vi "Measurement UI.vi"() -> ()   [LabVIEW 2021, in "ImageRendering.lvlib"]
uses:
  ImageRendering.lvlib
  <vilib>/vision/Image Controls.llb/IMAQ Image.ctl
  nivision.dll
  nivissvc.dll
panel:
  out "Average Time to receive image frame":dbl
  out "Time taken to receive image frame":dbl
  out "Image Acq time":string
  out "Display Frames per Second (approx)":u32
  out "Last Buffer Number":u32
  out "Time to convert back to Image (s)":dbl
  in  "Border Size":i32=3
  in  "Image Name":string="copy"
  in  "Image Type":u32(ring)=4 items=["Grayscale (U8)", "Grayscale (I16)", "Grayscale (SGL)", "Complex (CSG)", "RGB (U32)", "HSL (U32)", "RGB (U64)", "Grayscale (U16)"]
  out "Image Resolution":i32[](array[numeric])
  in  "Camera name":string
  out "Image Pixels (U32)":u32[](array[numeric])
  in  "Image Pixels (U64) 2":T1[][](array[typedef])
  in  "Image Converison Type":string(combo)="ImagePixelArray"
  out "Image Data Received":string
  out "value":u32[][](array[numeric])
  out "Image":T2(plugin-control)
  out "error out":errorcluster
  out "Image Data":string
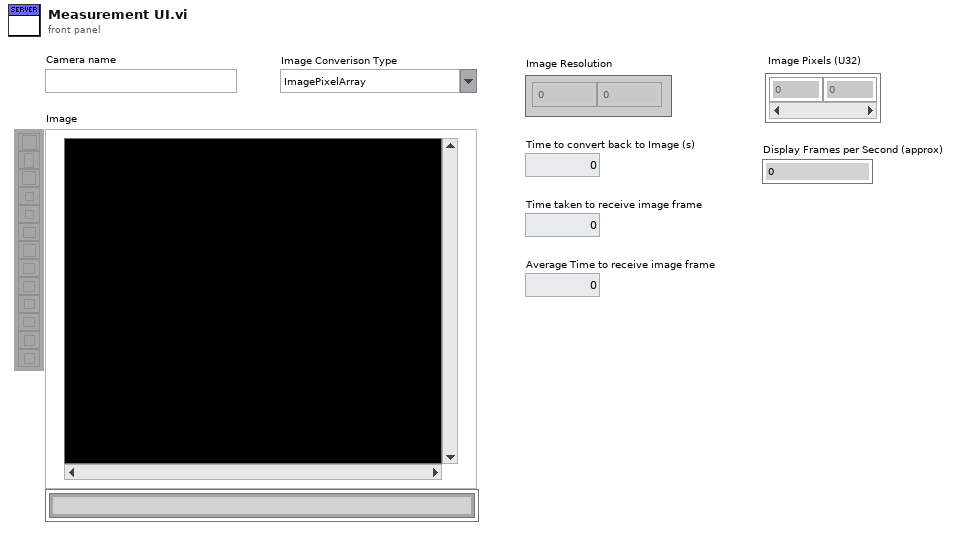
[diagram p1: front panel]
types:
  T1 = typedef "Color (U64)" = cluster{"Plane 3 (Blue)":u16, "Plane 2 (Green)":u16, "Plane 1 (Red)":u16, "Plane 4 (alpha)":u16}
  T2 = typedef "IMAQ Image.ctl" = refnum<image>
  T3 = cluster{"New Image":T2, "Run start time":timestamp, "Last Buffer Number":u32, "Time to receive image":dbl[]}
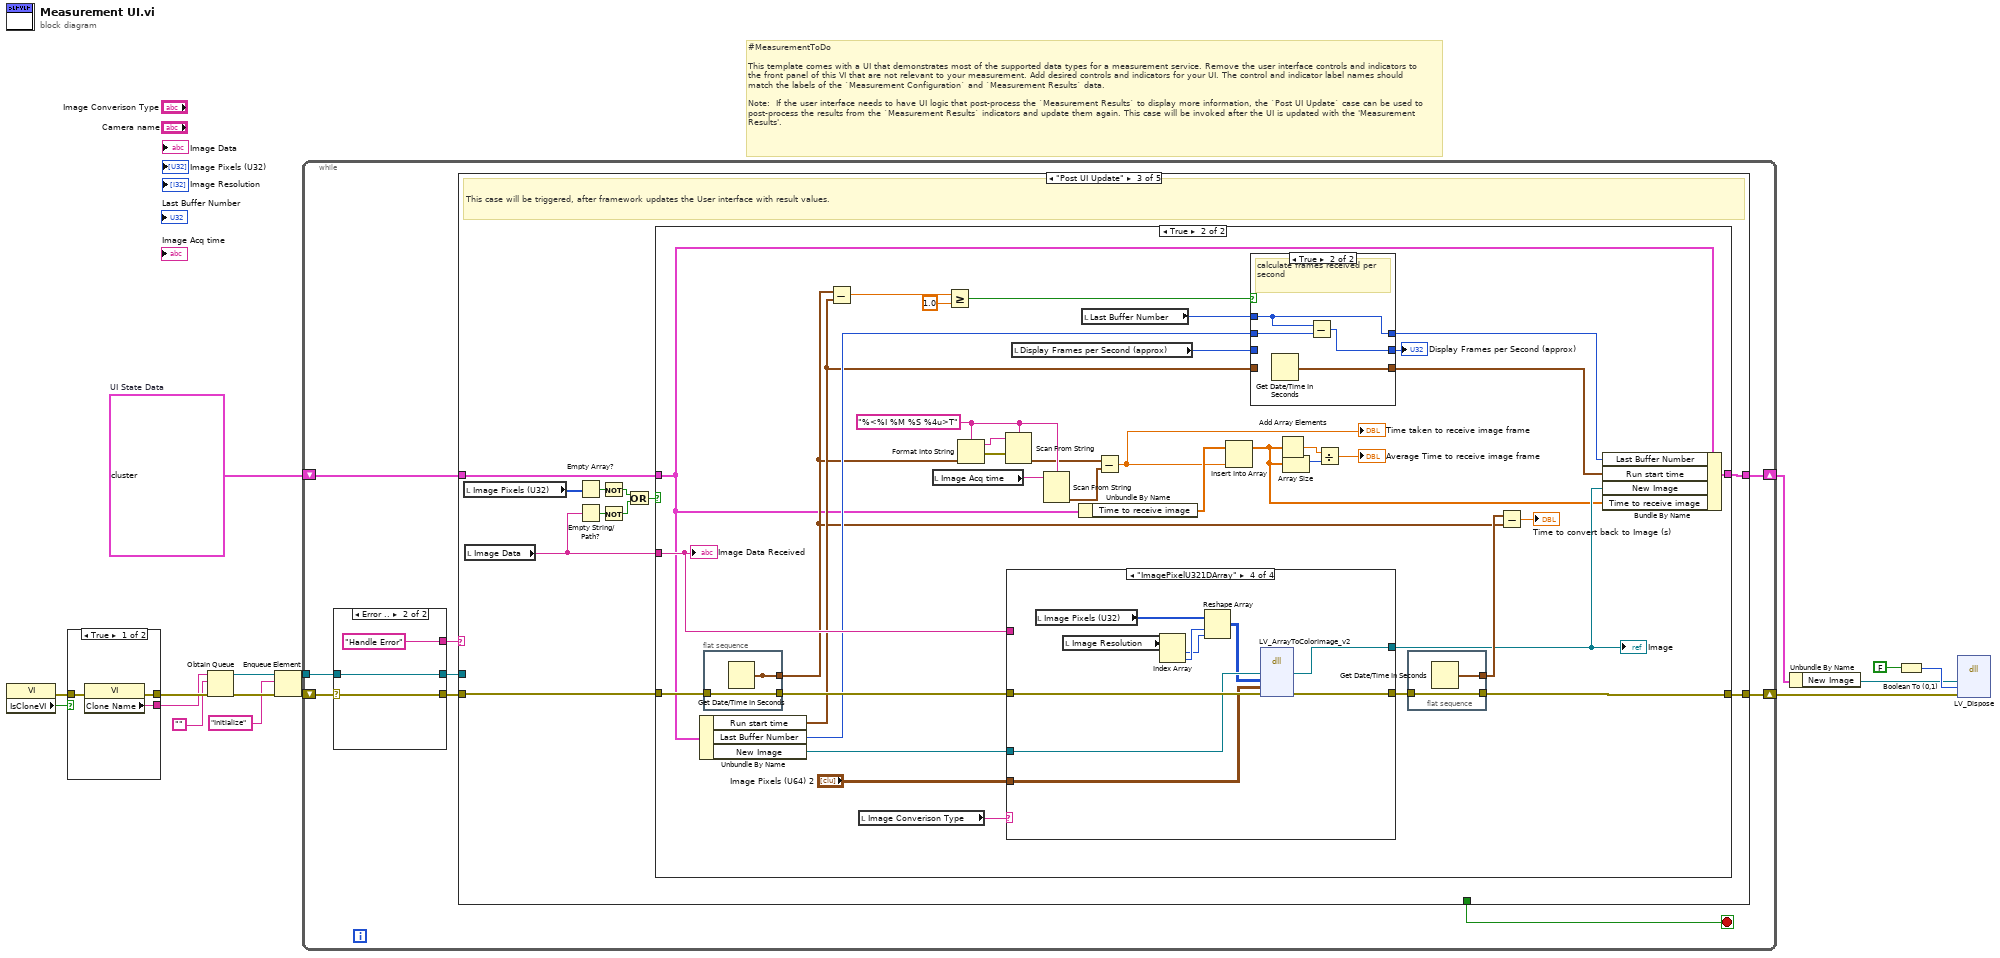
[diagram p0: block diagram]
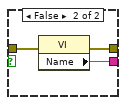
[diagram p2: hidden frame]
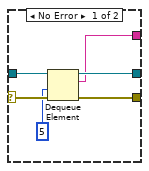
[diagram p3: hidden frame]
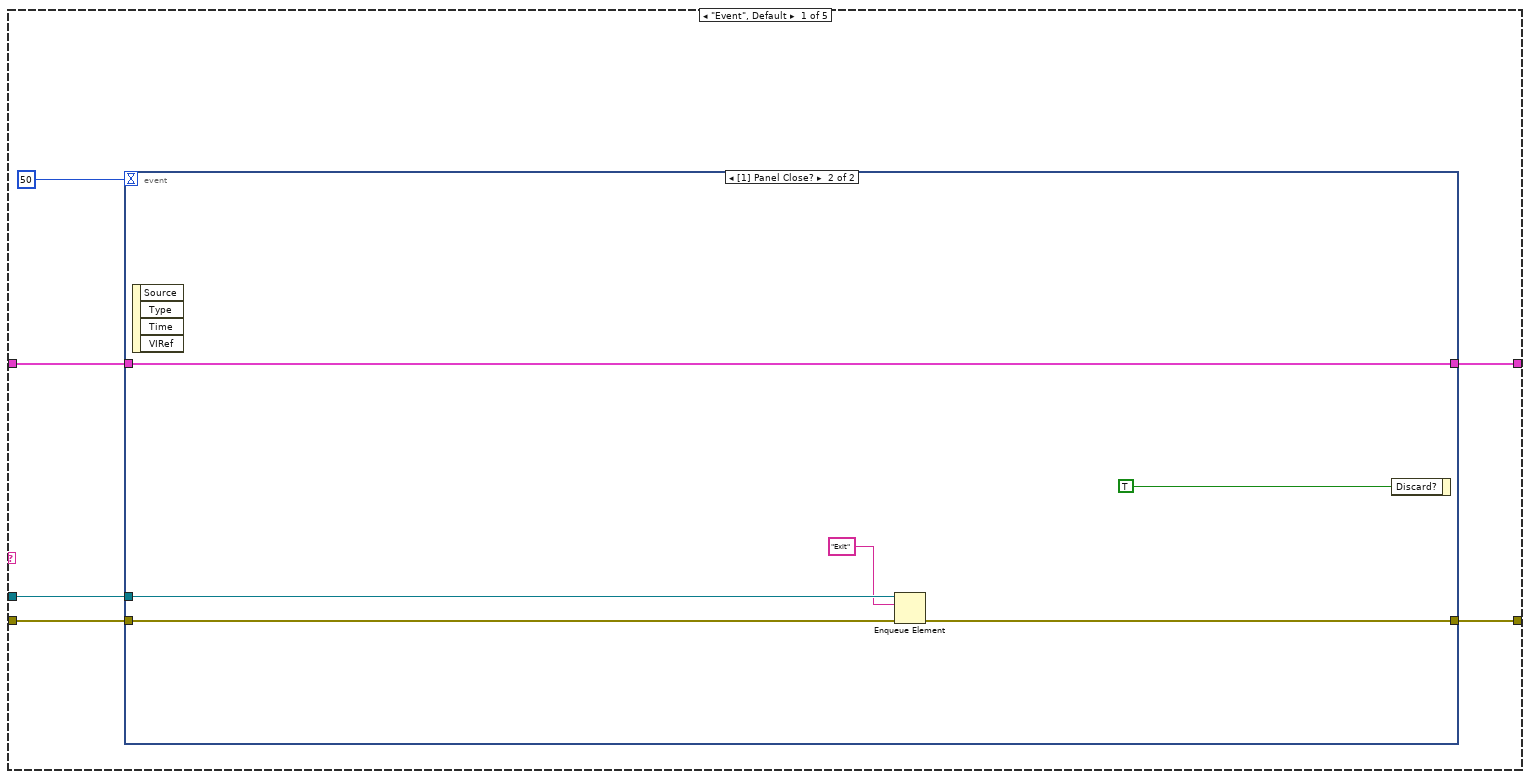
[diagram p4: hidden frame]
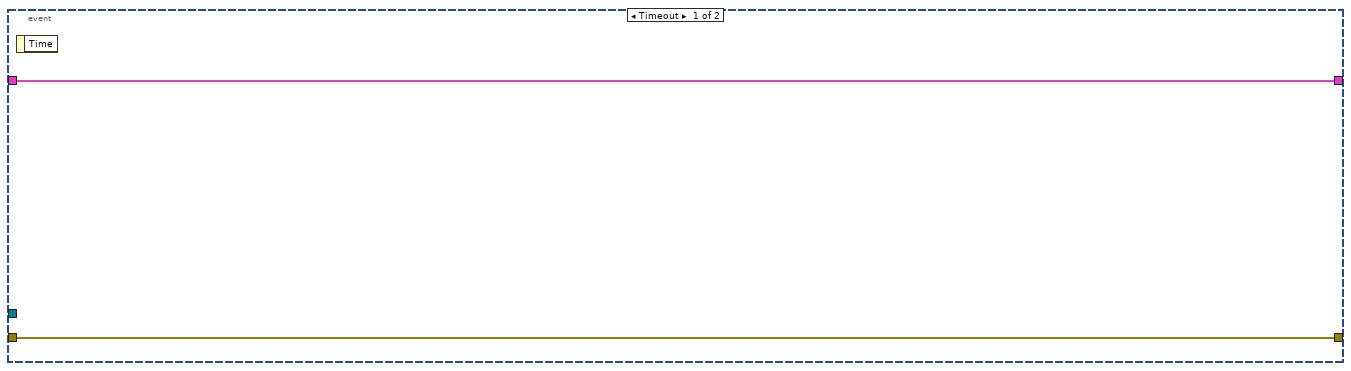
[diagram p5: hidden frame]
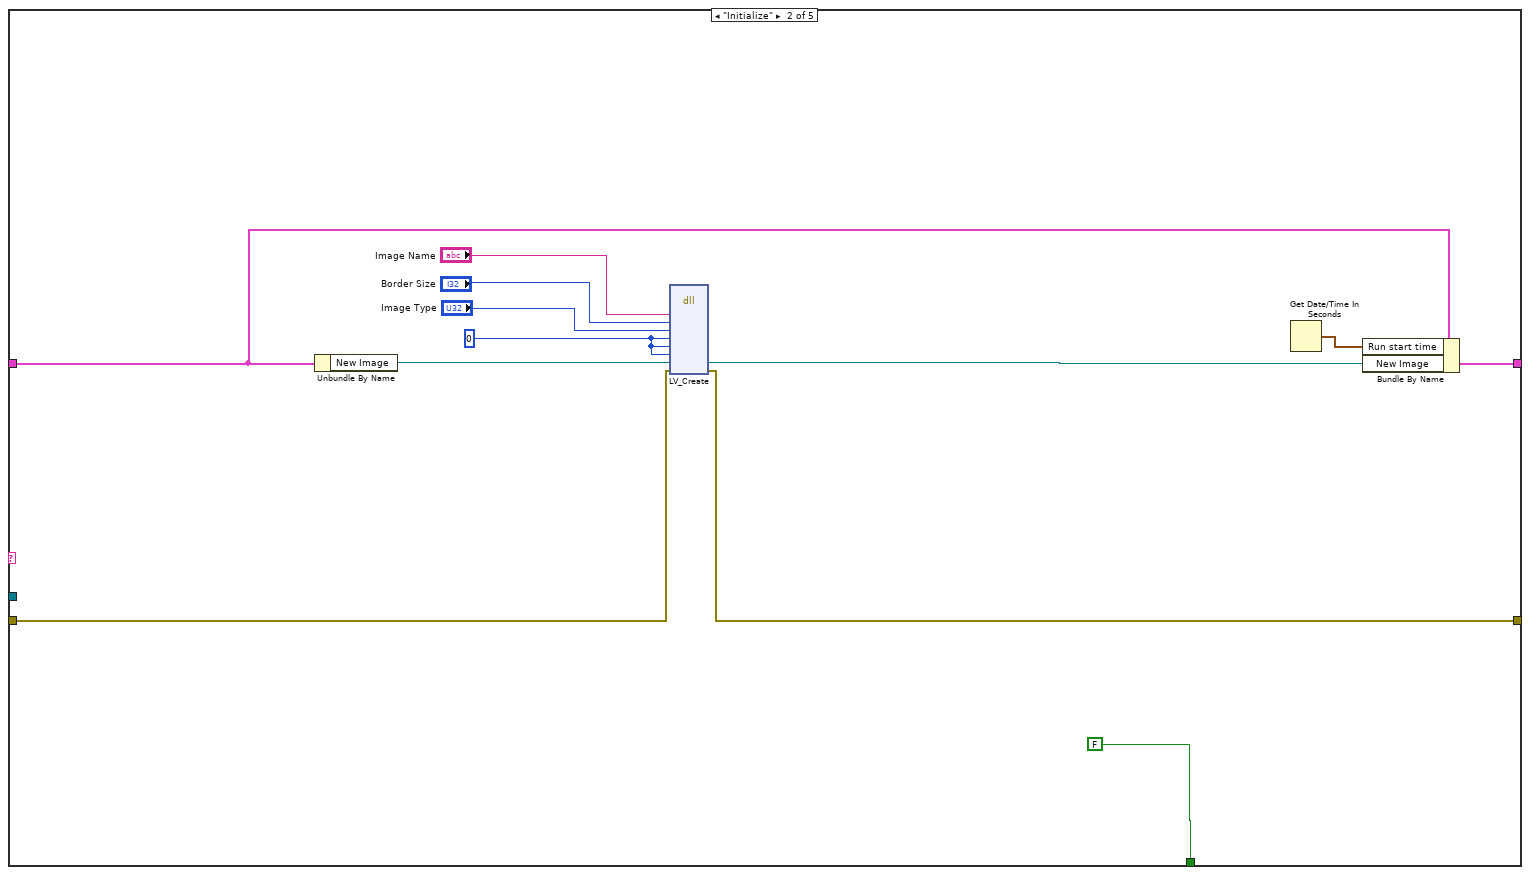
[diagram p6: hidden frame]
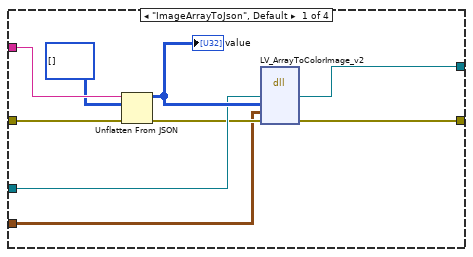
[diagram p9: hidden frame]
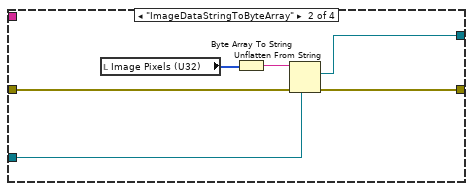
[diagram p10: hidden frame]
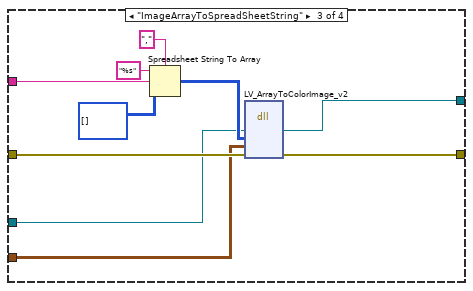
[diagram p11: hidden frame]
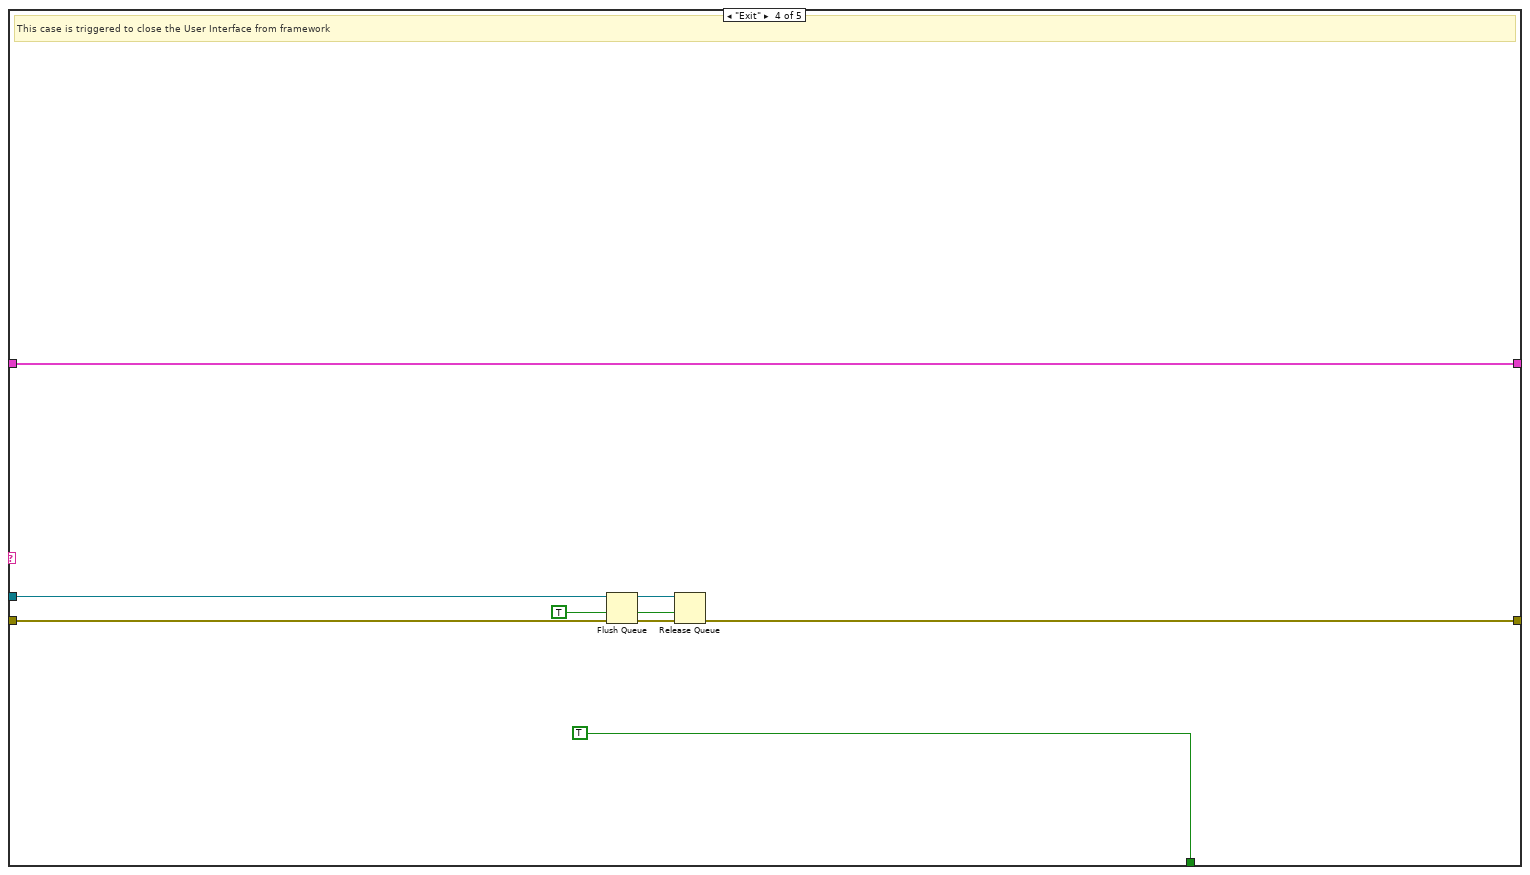
[diagram p12: hidden frame]
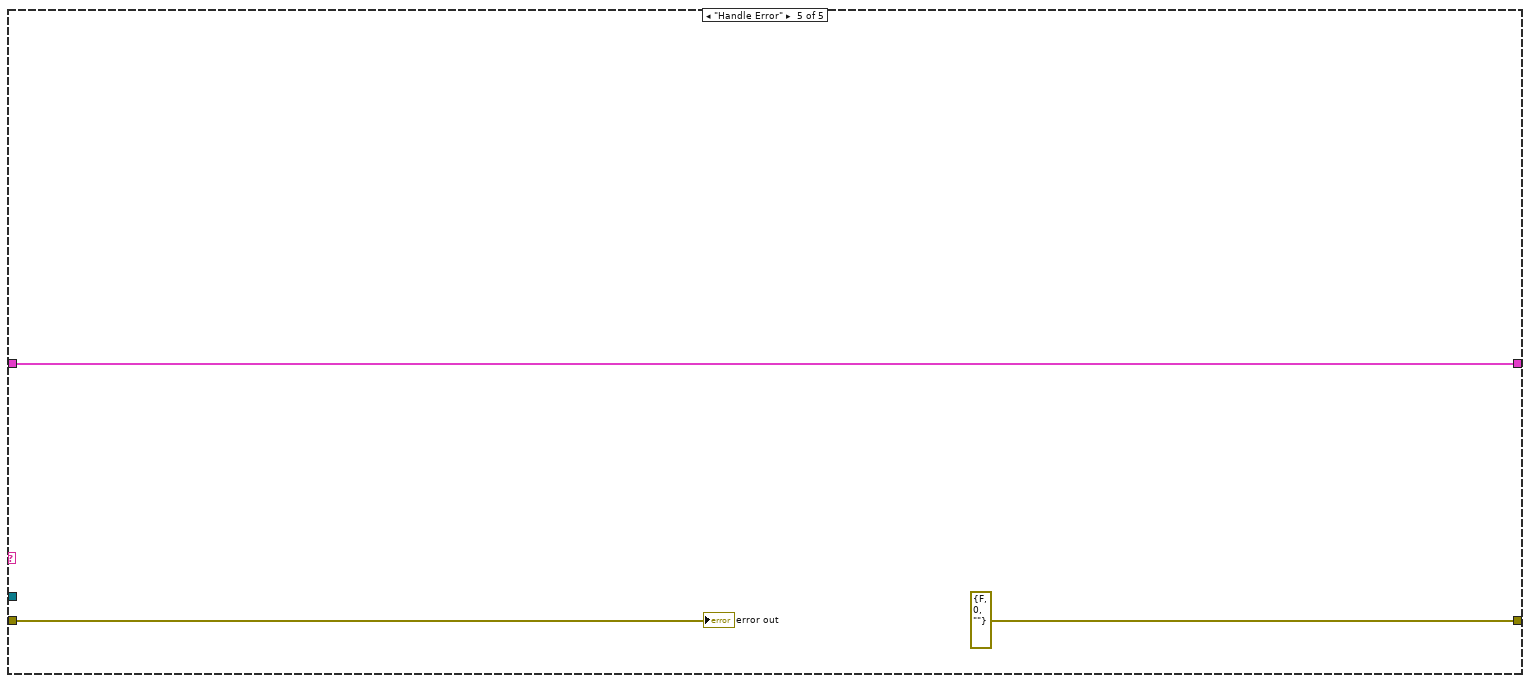
[diagram p13: hidden frame]
diagram:
  w2 = T3 {"New Image"=refnum, "Run start time"=timestamp(0 s since 1904-01-01), "Last Buffer Number"=0, "Time to receive image"=[]}  # UI State Data
  # "#MeasurementToDo  \n\nThis template comes with a UI that demonstrates most of the supported data types for a measurement service. Remove the user interface controls and indicators to the front panel of this VI that are not relevant to your measurement. Add desired controls and indicators for your UI. The control and indicator label names should match the labels of the `Measurement Configuration` and `Measurement Results` data.\n\nNote:  If the user interface needs to have UI logic that post-process the `Measurement Results` to display more information, the `Post UI Update` case can be used to post-process the results from the `Measurement Results` indicators and update them again. This case will be invoked after the UI is updated with the 'Measurement Results'."
  n1 = property class="VI"() -> (error out=w7:errorcluster, "IsCloneVI"=w8:bool)  [unwired: 2 in, 1 out]
  n2 = case shown="True" w8 {
    tunnel: [w19 w22] -> w16
    tunnel: [w18 w21] -> w15
    tunnel: w7 -> [w17 w20]
    frame True {
      n3 = property class="VI"(error in=w17) -> (error out=w19:errorcluster, "Clone Name"=w18:string)  [unwired: 1 in, 1 out]
    }
    frame False {
      n4 = property class="VI"(error in=w20) -> (error out=w22:errorcluster, "Name"=w21:string)  [unwired: 1 in, 1 out]
    }
  }
  n5 = Obtain Queue(name (unnamed)=w15, element data type="", error in (no error)=w16) -> (queue out=w12:refnum<queue>, error out=w14:errorcluster)  [unwired: 2 in, 1 out]
  n6 = Enqueue Element(queue=w12, element="Initialize", error in (no error)=w14) -> (queue out=w11:refnum<queue>, error out=w13:errorcluster)  [unwired: 1 in, 1 out]
  n7 = while {
    shift-right: [w27] -> w5
    shift-left: w13 -> [w31]
    tunnel: w11 -> [w30]
    shift-right: [w24] -> w3
    shift-left: w2 -> [w23]
    stop <- w26 stop-if-true
    n8 = case shown="Error .." w31 {
      selector: w31 -> [w37 w40]
      tunnel: [w36 w40] -> w25
      tunnel: w30 -> [w35 w39]
      tunnel: [w34 w39] -> w29
      tunnel: [w33 "Handle Error"] -> w28
      frame No Error {
        n9 = Dequeue Element(queue=w35, timeout in ms (-1)=5, error in (no error)=w37) -> (queue out=w34:refnum<queue>, element=w33:string, error out=w36:errorcluster)  [unwired: 1 out]
      }
      frame Error {
      }
    }
    n10 = case shown="\"Post UI Update\"" w28 {
      tunnel: w25 -> [w45 w61 w76 w169 w172]
      tunnel: w29 -> [w43 _ _ w167 _]
      tunnel: [w46 w55 w77 w164 errorcluster {"status"=FALSE, "code"=0, "source"=""} ("error out")] -> w27
      tunnel: [_ FALSE _ TRUE _] -> w26
      tunnel: [w41 w58 w68 w162 w171] -> w24
      tunnel: w23 -> [w42 w57 w67 w162 w171]
      frame "Event", Default {
        n11 = event shown="[1] Panel Close?" {
          selector: _ -> [_ _]
          dyn-events: _ -> [_ _]
          timeout: 50 -> [_ _]
          tunnel: [w48 w52] -> w46
          tunnel: w45 -> [w48 w53]
          tunnel: w43 -> [_ w51]
          tunnel: w42 -> [w47 w49]
          tunnel: [w47 w49] -> w41
          event Timeout {
            n12 = event-data() -> ()  [unwired: 1 in, 1 out]
          }
          event Panel Close? {
            n13 = event-data() -> ()  [unwired: 1 in, 4 out]
            n14 = Enqueue Element(queue=w51, element="Exit", error in (no error)=w53) -> (error out=w52:errorcluster)  [unwired: 1 in, 2 out]
            n15 = event-data("Discard?"=TRUE) -> ()  [unwired: 1 in, 1 out]
          }
        }
      }
      frame "Initialize" {
        w62 = 0
        n16 = Unbundle By Name(w57) -> ("New Image"=w59:T2)
        n17 = dll-call lib="nivissvc.*" fn="LV_Create"("name"="Image Name", "border"="Border Size", "imageType"="Image Type", "width"=w62, "height"=w62, "lock space"=w62, "image"=w59, "error out 2"=w61) -> ("image"=w60:T2, "error out 2"=w55:errorcluster)  [unwired: 9 in, 3 out]
        n18 = Get Date/Time In Seconds() -> (seconds since 1Jan1904=w56:timestamp)
        n19 = Bundle By Name(cluster=w57, "Run start time"=w56, "New Image"=w60) -> (w58:T3)
      }
      frame "Post UI Update" {
        # "This case will be triggered, after framework updates the User interface with result values."
        n20 = local read "Image Pixels (U32)"() -> (w74:u32[])
        n21 = local read "Image Data"() -> (w72:string)
        n22 = Empty Array?(array=w74) -> (empty?=w75:bool)
        n23 = Empty String/Path?(string/path=w72) -> (empty?=w71:bool)
        n24 = Not(x=w75) -> (.not. x?=w73:bool)
        n25 = Not(x=w71) -> (.not. x?=w70:bool)
        n26 = Or(x=w73, y=w70) -> (x .or. y?=w69:bool)
        n27 = case shown="True" w69 {
          tunnel: [w79 w110] -> w77
          tunnel: w76 -> [w79 w114]
          tunnel: w72 -> [_ w112]
          tunnel: [w78 w106] -> w68
          tunnel: w67 -> [w78 w83]
          frame False {
          }
          frame True {
            w93 = "%<%I %M %S %4u>T" ("format string")
            n28 = Unbundle By Name(w83) -> ("Run start time"=w99:timestamp, "Last Buffer Number"=w101:u32, "New Image"=w87:T2)
            n29 = flat-sequence {
              tunnel: w114 -> [w159]
              tunnel: [w159] -> w109
              tunnel: [w158] -> _
              tunnel: [w158] -> w88
              frame #0 {
                n30 = Get Date/Time In Seconds() -> (seconds since 1Jan1904=w158:timestamp)
              }
            }
            n31 = Subtract(x=w88, y=w99) -> (x-y=w105:dbl)
            n32 = local read "Image Converison Type"() -> (w113:string)
            n33 = local read "Image Acq time"() -> (w97:string)
            n34 = Greater Or Equal?(x=w105, y=1.0) -> (x >= y?=w103:bool)
            n35 = Format Into String(format string=w93, w88) -> (resulting string=w94:string, error out=w95:errorcluster)  [unwired: 2 in]
            n36 = Scan From String(format string=w93, input string=w94, error in=w95) -> (output 1=w92:timestamp)  [unwired: 2 in, 3 out]
            n37 = case shown="\"ImagePixelU321DArray\"" w113 {
              tunnel: w112 -> [w131 _ w147 _]
              tunnel: w87 -> [w128 w135 w140 w155]
              tunnel: [w127 w134 w139 w154] -> w86
              tunnel: [w126 w136 w143 w156] -> w115
              tunnel: w109 -> [w125 w137 w144 w157]
              tunnel: "Image Pixels (U64) 2" -> [w123 _ w138 w153]
              frame "ImageArrayToJson", Default {
                n38 = Unflatten From JSON(JSON string=w131, type and defaults=u32[][] [] ("Image Pixels (U32)"), error in (no error)=w125) -> (value=w129:u32[][], error out=w124:errorcluster)  [unwired: 4 in]
                "value" <- w129
                n39 = dll-call lib="nivision.*" fn="LV_ArrayToColorImage_v2"("image"=w128, "array32"=w129, "array64"=w123, "error"=w124) -> ("image"=w127:T2, "error"=w126:errorcluster)  [unwired: 5 in, 3 out]
              }
              frame "ImageDataStringToByteArray" {
                n40 = local read "Image Pixels (U32)"() -> (w133:u32[])
                n41 = Byte Array To String(unsigned byte array=w133) -> (string=w132:string)
                n42 = Unflatten From String(type=w135, binary string=w132, error in (no error)=w137) -> (value=w134:T2, error out=w136:errorcluster)  [unwired: 2 in, 1 out]
              }
              frame "ImageArrayToSpreadSheetString" {
                n43 = Spreadsheet String To Array(delimiter (Tab)=",", format string="%s", spreadsheet string=w147, array type (2D Dbl)=u32[][] [] ("Image Pixels (U32)")) -> (array=w142:u32[][])
                n44 = dll-call lib="nivision.*" fn="LV_ArrayToColorImage_v2"("image"=w140, "array32"=w142, "array64"=w138, "error"=w144) -> ("image"=w139:T2, "error"=w143:errorcluster)  [unwired: 5 in, 3 out]
              }
              frame "ImagePixelU321DArray" {
                n45 = local read "Image Pixels (U32)"() -> (w152:u32[])
                n46 = local read "Image Resolution"() -> (w151:i32[])
                n47 = Index Array(array=w151) -> (element #1=w149:i32, element #2=w150:i32)  [unwired: 2 in]
                n48 = Reshape Array(w152, w150, w149) -> (w148:u32[][])
                n49 = dll-call lib="nivision.*" fn="LV_ArrayToColorImage_v2"("image"=w155, "array32"=w148, "array64"=w153, "error"=w157) -> ("image"=w154:T2, "error"=w156:errorcluster)  [unwired: 5 in, 3 out]
              }
            }
            "Image" <- w86
            n50 = local read "Display Frames per Second (approx)"() -> (w100:u32)
            n51 = Scan From String(format string=w93, input string=w97) -> (output 1=w96:timestamp)  [unwired: 3 in, 3 out]
            n52 = Unbundle By Name(w83) -> ("Time to receive image"=w82:dbl[])
            n53 = local read "Last Buffer Number"() -> (w102:u32)
            n54 = Subtract(x=w92, y=w96) -> (x-y=w81:dbl)
            "Time taken to receive image frame" <- w81
            n55 = Insert Into Array(array=w82, new element=w81) -> (w80:dbl[])  [unwired: 1 in]
            n56 = case shown="True" w103 {
              tunnel: w101 -> [w116 w122]
              tunnel: [w118 w121] -> w84
              tunnel: w99 -> [w118 _]
              tunnel: [w117 w120] -> w98
              tunnel: w100 -> [w117 _]
              tunnel: w102 -> [_ w119]
              tunnel: [w116 w119] -> w85
              frame False {
              }
              frame True {
                # "calculate frames received per second"
                n57 = Get Date/Time In Seconds() -> (seconds since 1Jan1904=w121:timestamp)
                n58 = Subtract(x=w119, y=w122) -> (x-y=w120:u32)
              }
            }
            "Display Frames per Second (approx)" <- w98
            n59 = Add Array Elements(numeric array=w80) -> (sum=w91:dbl)
            n60 = Array Size(array=w80) -> (size(s)=w90:i32)
            n61 = Divide(x=w91, y=w90) -> (x/y=→"Average Time to receive image frame":dbl)
            n62 = flat-sequence {
              tunnel: w115 -> [w161]
              tunnel: [w161] -> w110
              tunnel: [w160] -> w108
              frame #0 {
                n63 = Get Date/Time In Seconds() -> (seconds since 1Jan1904=w160:timestamp)
              }
            }
            n64 = Subtract(x=w108, y=w88) -> (x-y=→"Time to convert back to Image (s)":dbl)
            n65 = Bundle By Name(cluster=w83, "Last Buffer Number"=w85, "Run start time"=w84, "New Image"=w86, "Time to receive image"=w80) -> (w106:T3)
            "Image Data Received" <- w112
          }
        }
      }
      frame "Exit" {
        # "This case is triggered to close the User Interface from framework"
        n66 = Flush Queue(queue=w167, error in (no error)=w169) -> (queue out=w166:refnum<queue>, error out=w165:errorcluster)  [unwired: 1 out]
        n67 = Release Queue(queue=w166, force destroy? (F)=TRUE, error in (no error)=w165) -> (error out=w164:errorcluster)  [unwired: 2 out]
      }
      frame "Handle Error" {
        "error out" <- w172
      }
    }
  }
  n68 = Unbundle By Name(w3) -> ("New Image"=w1:T2)
  n69 = Boolean To (0,1)(Boolean=FALSE) -> (0, 1=w6:i16)
  n70 = dll-call lib="nivissvc.*" fn="LV_Dispose"("image"=w1, "disposeAll"=w6, "err"=w5) -> ()  [unwired: 5 in, 4 out]
